vi "GetPersistentConfiguration.vi"(8 "ErrorIn":errorcluster, 9 "DataIn":variant, 11 "ReferenceIn":refnum<class "TemplateGUI.lvclass">) -> (0 "ErrorOut":errorcluster, 1 "DataOut":variant, 3 "ReferenceOut":refnum<class "TemplateGUI.lvclass">)   [LabVIEW 2021, in "TemplateGUIOpenGDSActiveObject.lvlib" / "TemplateGUI.lvclass"]
doc: "Retrieve the persistent data of the object. For TAF these are stored in the attributes of the variant"
uses:
  TemplateGUI.lvclass
  Library_TAF_ApplicationFramework/TAFBaseGUI/TAFBaseGUI.lvclass
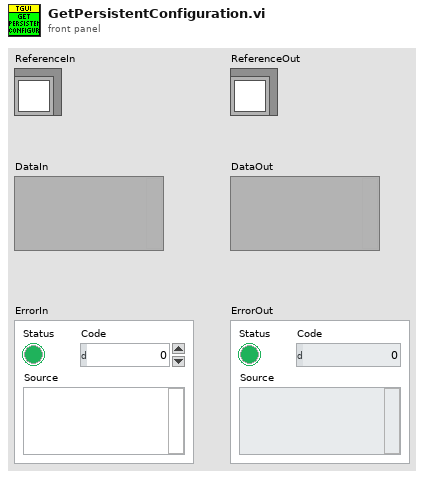
[diagram p1: front panel]
types:
  T1 = typedef "TemplateGUIOpenGDSActiveObject.lvlib/TemplateGUI.lvclass/ObjectAttributes.ctl" = cluster{"Interfaces":cluster{"Dummys":refnum<class>}, "Locals":cluster{"MainGUIActive":refnum<queue>}, "Persistent":cluster{"Dummy":bool}}
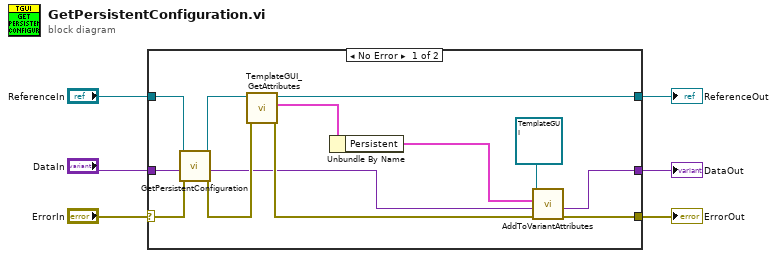
[diagram p0: block diagram]
diagram:
  n1 = case shown="No Error" "ErrorIn" {
    selector: "ErrorIn" -> [w19 w22]
    tunnel: [w17 w22] -> w5
    tunnel: [w14 w21] -> w3
    tunnel: "ReferenceIn" -> [w10 w21]
    tunnel: [w13 w20] -> w2
    tunnel: "DataIn" -> [w8 w20]
    frame No Error {
      n2 = call-parent "GetPersistentConfiguration.vi"("ErrorIn"=w19, "DataIn"=w8, "ReferenceIn"=w10) -> ("ErrorOut"=w16:errorcluster, "DataOut"=w7:variant, "ReferenceOut"=w9:refnum<class "TemplateGUI.lvclass">)  [unwired: 6 in]
      n3 = call "TemplateGUI_GetAttributes.vi"("ErrorIn"=w16, "ReferenceIn"=w9) -> ("ErrorOut"=w18:errorcluster, "Data"=w15:T1, "ReferenceOut"=w14:refnum<class "TemplateGUI.lvclass">)  [unwired: 6 in, 1 out]
      n4 = Unbundle By Name(w15) -> ("Persistent"=w12:cluster{"Dummy":bool})
      n5 = call "AddToVariantAttributes.vi"("ErrorIn"=w18, "DataInIn"=w7, "PersistentData"=w12, "Object"=refnum<class "TemplateGUI.lvclass"> refnum ("VerticalButtonBar")) -> ("ErrorOut"=w17:errorcluster, "DataInOut"=w13:variant)  [unwired: 6 in]
    }
    frame Error {
    }
  }
  "ErrorOut" <- w5
  "ReferenceOut" <- w3
  "DataOut" <- w2
